vi "Main.vi"() -> ()   [LabVIEW 2018]
uses:
  Typedefs/States.ctl
  Typedefs/Element.ctl
  Typedefs/TestSequence.ctl
  C:/GIT/gaialabviewclient/Gaia_LabVIEW/Resources/JOT.GaiaClient.dll
  Resources/JOT.GaiaClient.dll
panel:
  out "error out":errorcluster
  in  "Exit":bool
  in  "Tab Control":enum32{"TestSequense", "ManualControls"}(tab)
  out "EventLog":string
  in  "StartTest":bool
  in  "DutLock":bool
  in  "BatteryConnector":bool
  # "StateApps"
  # "MainRobot"
  # "More StateApp manual controls \ncan be added here"
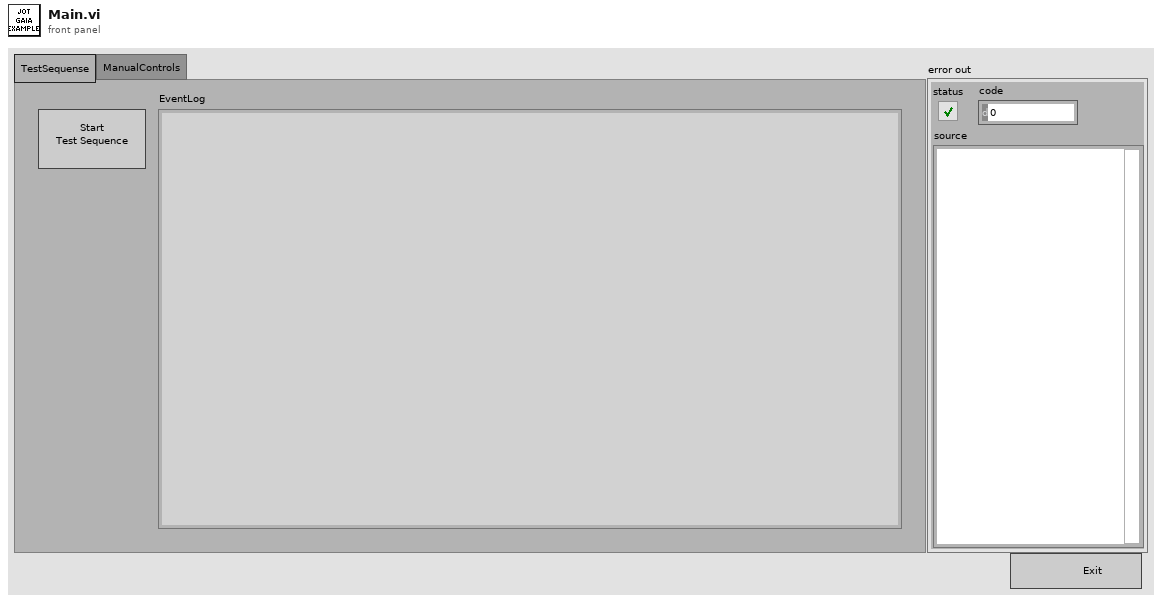
[diagram p1: front panel]
types:
  T1 = typedef "TestSequence.ctl" = enum16{"WaitDUT", "PreliminaryOperations", "WaitSlideClosed", "Test1", "ReleaseDUT"}
  T2 = typedef "Element.ctl" = cluster{"State":T3, "Application":string, "Action":string, "G code":string}
  T3 = typedef "States.ctl" = enum16{"InitGaiaClient", "Idle", "RobotManualCtr", "StateAppsManualCtr", "TestSequence", "Exit"}
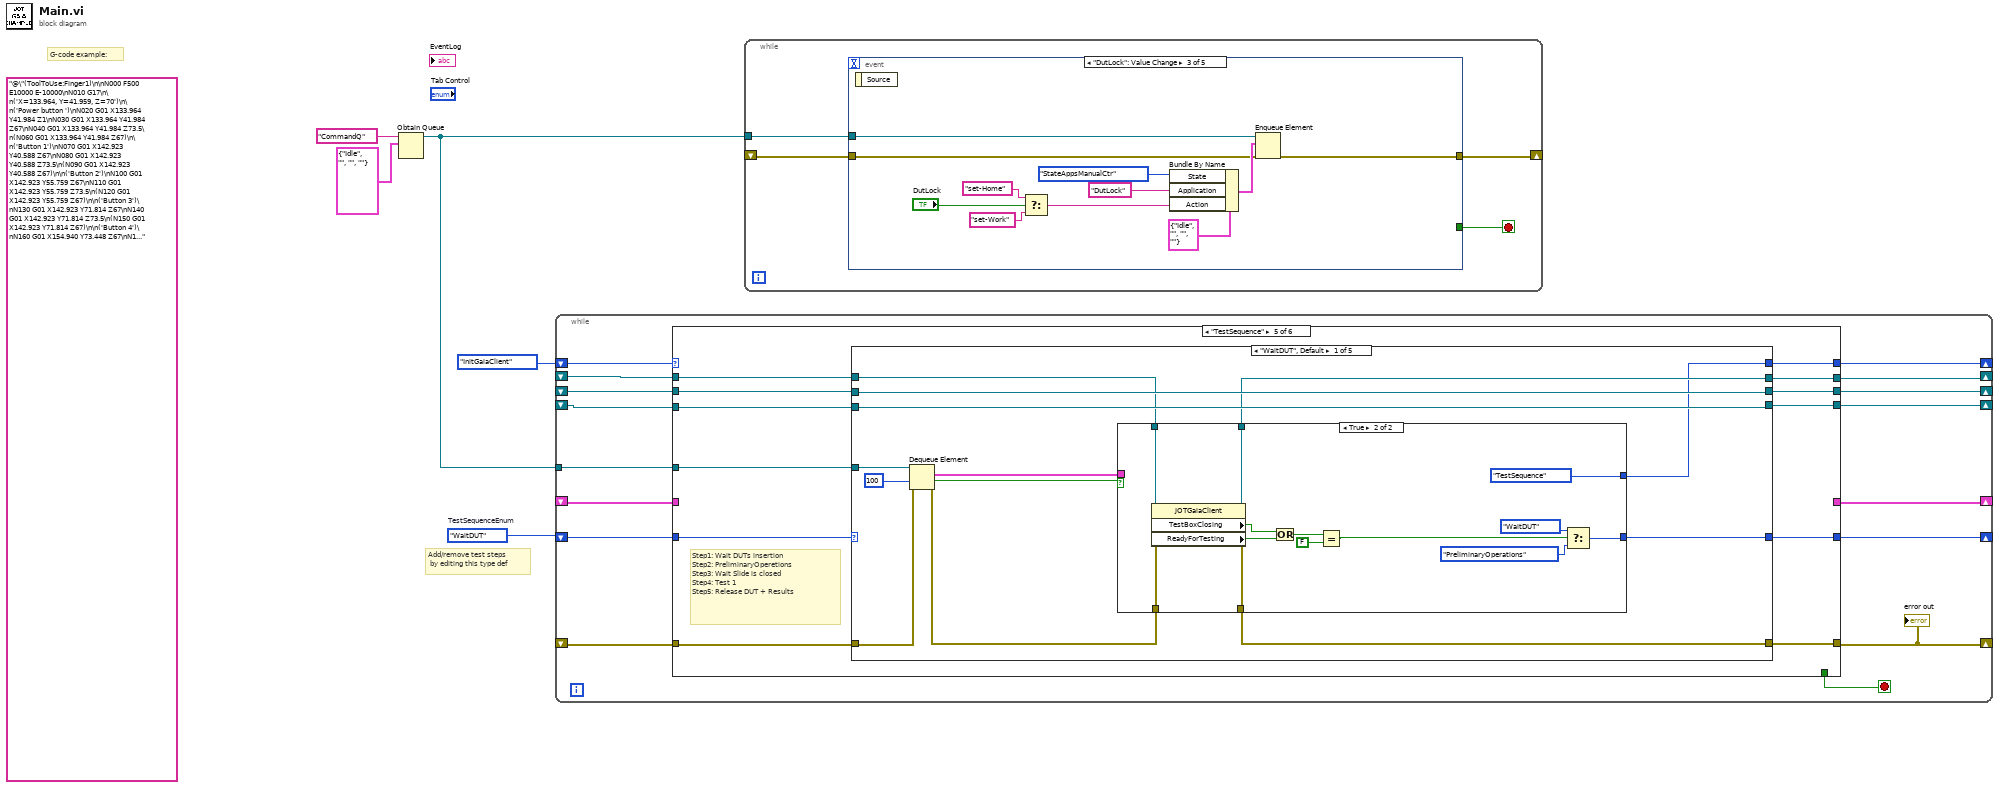
[diagram p0: block diagram]
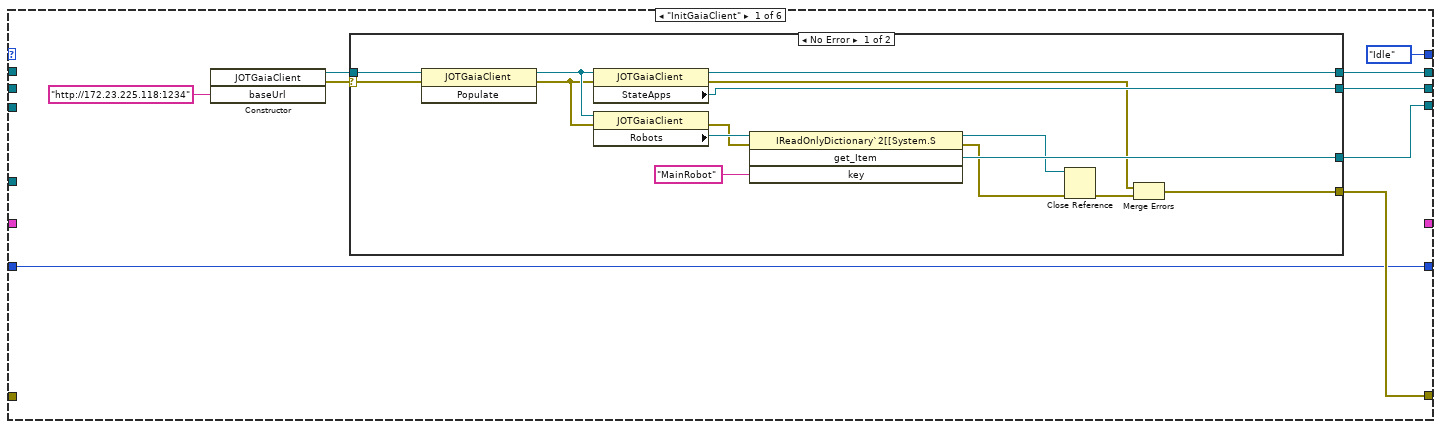
[diagram p2: hidden frame]
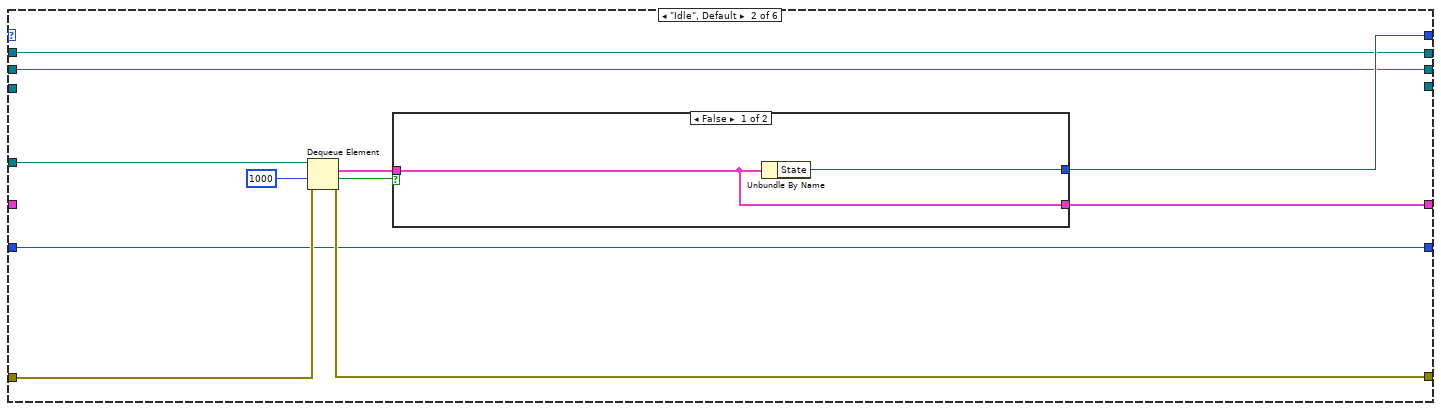
[diagram p4: hidden frame]
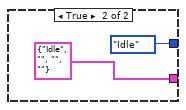
[diagram p5: hidden frame]
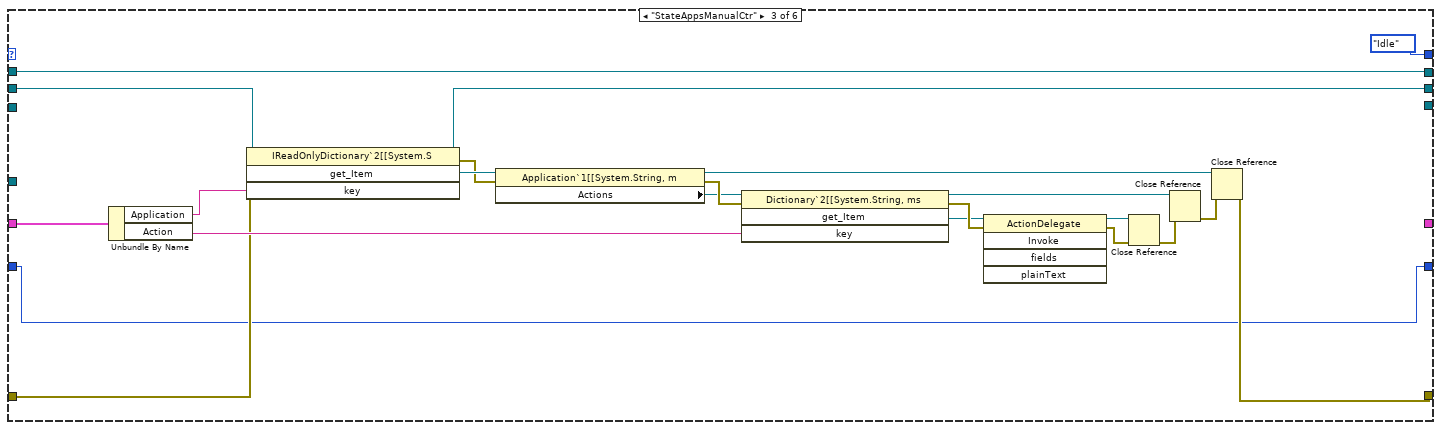
[diagram p6: hidden frame]
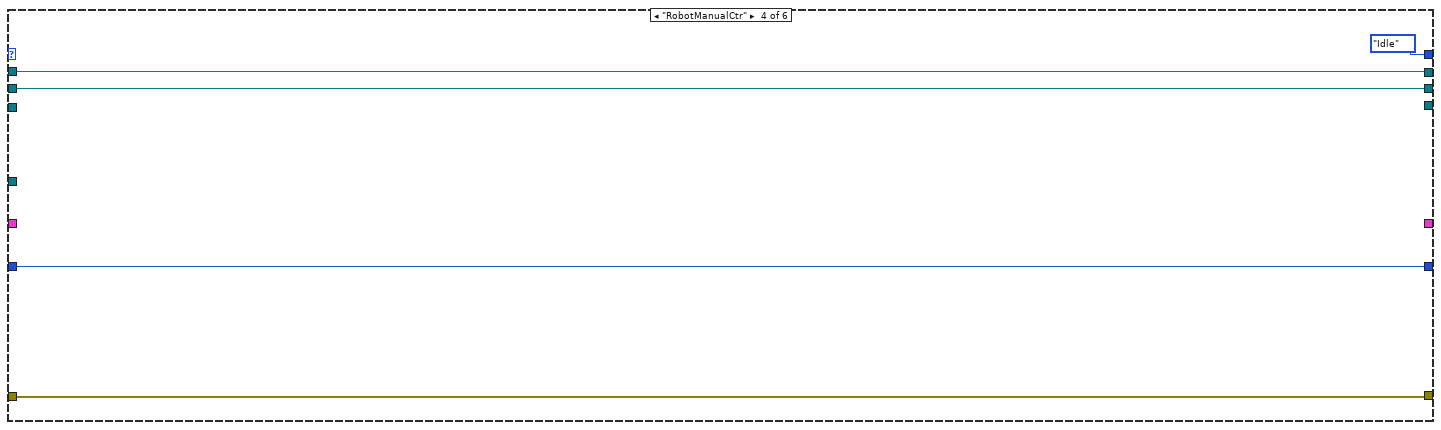
[diagram p7: hidden frame]
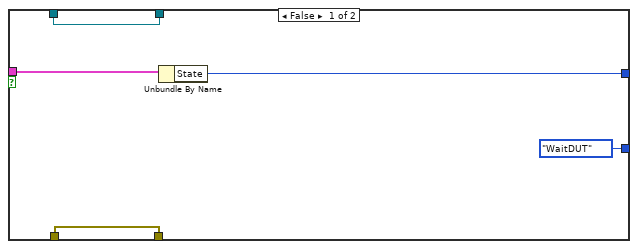
[diagram p8: hidden frame]
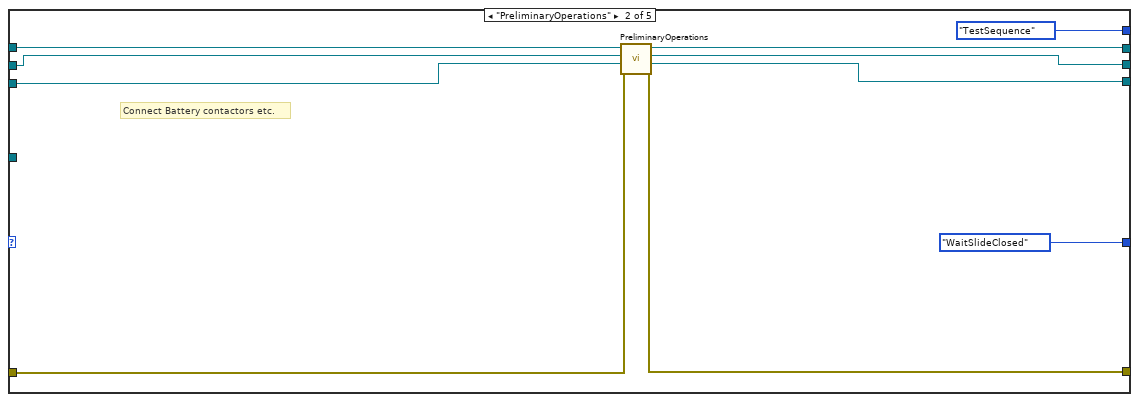
[diagram p9: hidden frame]
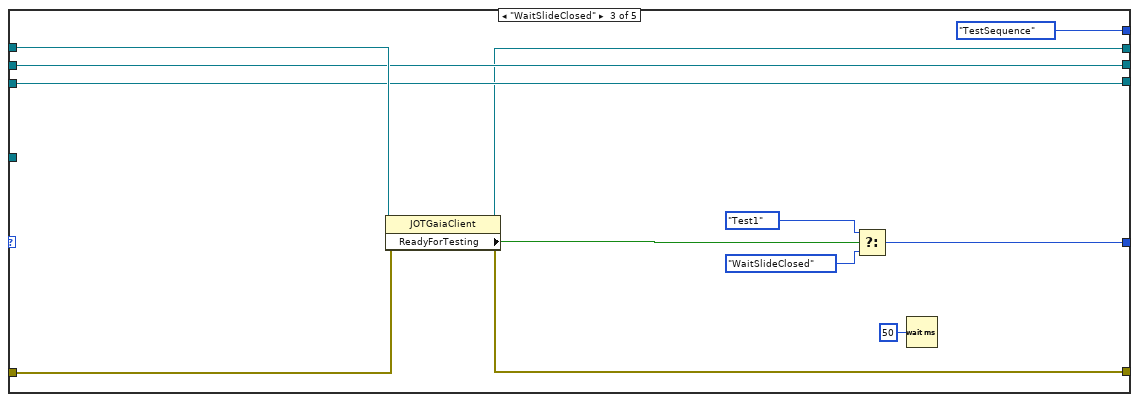
[diagram p10: hidden frame]
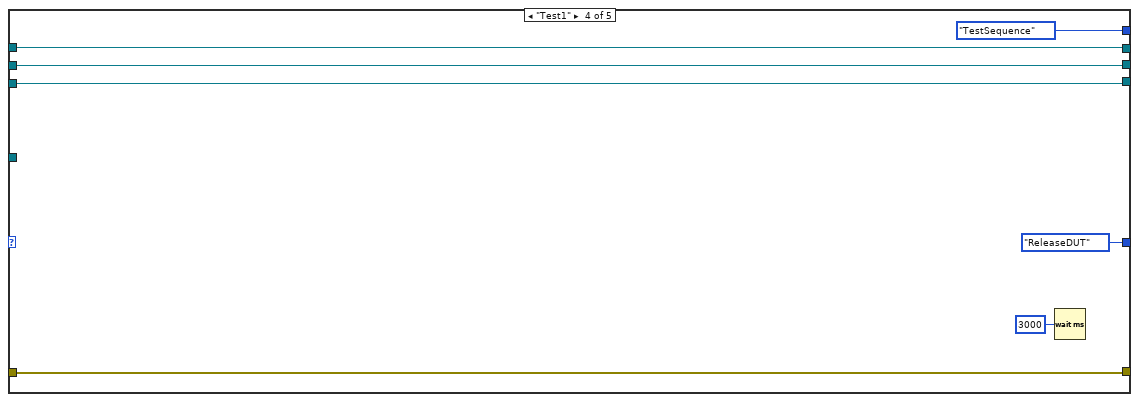
[diagram p11: hidden frame]
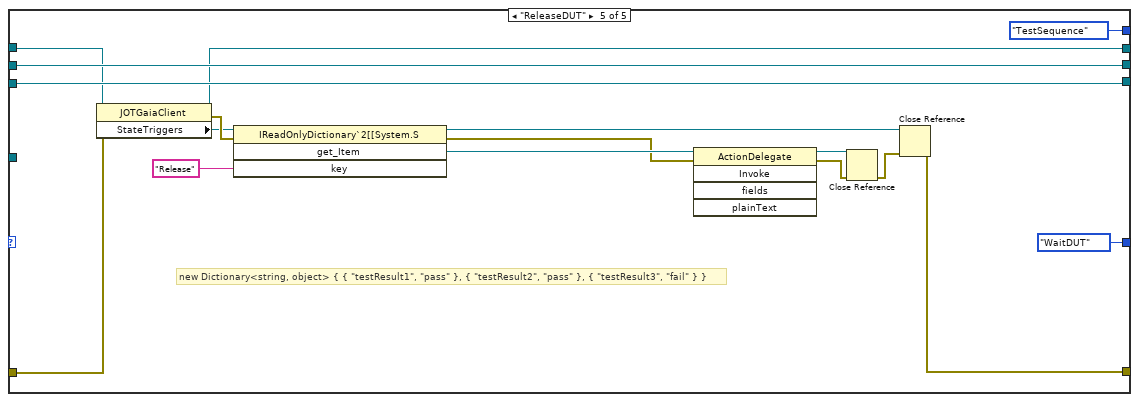
[diagram p12: hidden frame]
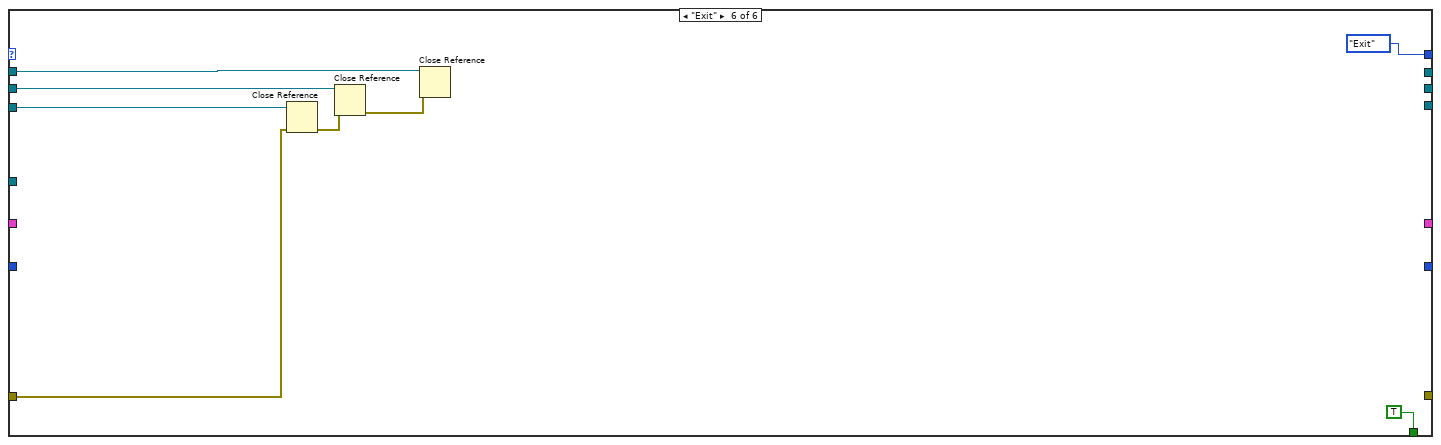
[diagram p13: hidden frame]
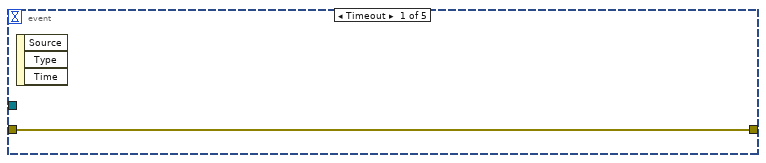
[diagram p14: hidden frame]
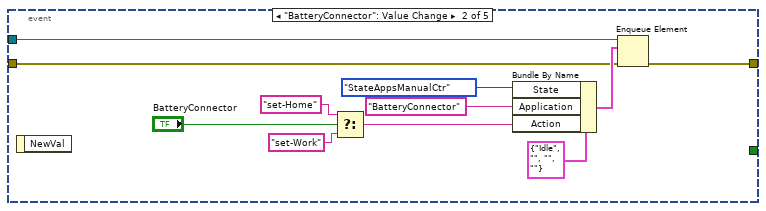
[diagram p15: hidden frame]
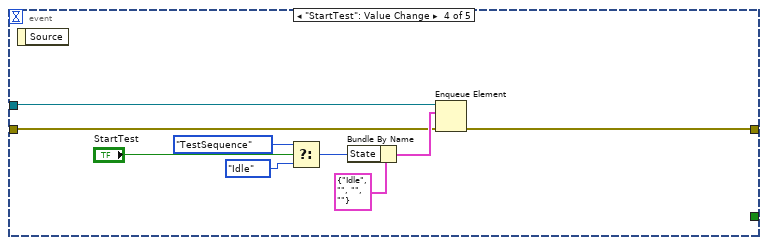
[diagram p16: hidden frame]
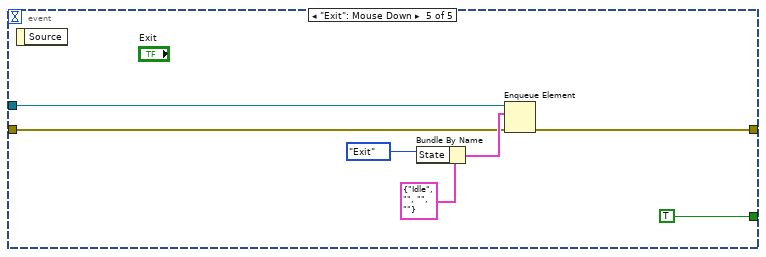
[diagram p17: hidden frame]
diagram:
  w1 = TestSequence."WaitDUT"  # TestSequenceEnum
  (unwired) "@\"(ToolToUse:Finger1)\n\nN000 F500 E10000 E-10000\nN010 G17\n\n('X=133.964, Y=41.959, Z=70')\n\n('Power button ')\nN020 G01 X133.964 Y41.984 Z1\nN030 G01 X133.964 Y41.984 Z67\nN040 G01 X133.964 Y41.984 Z73.5\n(N060 G01 X133.964 Y41.984 Z67)\n\n('Button 1')\nN070 G01 X142.923 Y40.588 Z67\nN080 G01 X142.923 Y40.588 Z73.5\n(N090 G01 X142.923 Y40.588 Z67)\n\n('Button 2')\nN100 G01 X142.923 Y55.759 Z67\nN110 G01 X142.923 Y55.759 Z73.5\n(N120 G01 X142.923 Y55.759 Z67)\n\n('Button 3')\nN130 G01 X142.923 Y71.814 Z67\nN140 G01 X142.923 Y71.814 Z73.5\n(N150 G01 X142.923 Y71.814 Z67)\n\n('Button 4')\nN160 G01 X154.940 Y73.448 Z67\nN170 G01 X154.940 Y73.448 Z73.5\n(N180 G01 X154.940 Y73.448 Z67)\n\n('Button 5')\nN190 G01 X154.940 Y55.778 Z67\nN200 G01 X154.940 Y55.778 Z73.2\n(N210 G01 X154.940 Y55.778 Z67)\n\n('Button 6')\nN220 G01 X154.940 Y38.754 Z67\nN230 G01 X154.940 Y38.754 Z73.5\n(N240 G01 X154.940 Y38.754 Z67)\n\n('Button 7')\nN250 G01 X167.756 Y42.098 Z67\nN260 G01 X167.756 Y42.098 Z73.2\n(N270 G01 X167.756 Y42.098 Z67)\n\n('Button 8')\nN280 G01 X167.756 Y55.883 Z67\nN290 G01 X167.756 Y55.883 Z73.3\n(N300 G01 X167.756 Y55.883 Z67)\n\n('Button 9')\nN310 G01 X167.756 Y69.886 Z67\nN320 G01 X167.756 Y69.886 Z73.2\n(N330 G01 X167.756 Y69.886 Z67)\""
  # "Add/remove test steps\n by editing this type def"
  # "G-code example:"
  n1 = Obtain Queue(name (unnamed)="CommandQ", element data type=T2 {"State"=enum."Idle", "Application"="", "Action"="", "G code"=""}) -> (queue out=w2:refnum<queue>)  [unwired: 3 in, 2 out]
  n2 = while {
    shift-right: [w14] -> _
    shift-left: States."InitGaiaClient" -> [w21]
    shift-right: [w20] -> _
    shift-left: _ -> [w9]
    shift-right: [w19] -> _
    shift-left: _ -> [w8]
    shift-right: [w16] -> _
    shift-left: _ -> [w17]
    shift-right: [w15] -> _
    shift-left: _ -> [w10]
    tunnel: w2 -> [w13]
    shift-right: [w12] -> _
    shift-left: _ -> [w11]
    shift-right: [w6] -> _
    shift-left: w1 -> [w7]
    stop <- w18 stop-if-true
    n3 = case shown="\"TestSequence\"" w21 {
      tunnel: [_ _ _ _ _ TRUE] -> w18
      tunnel: [w28 w48 w62 w85 w95 _] -> w20
      tunnel: [w27 w49 w69 w86 w94 _] -> w19
      tunnel: w17 -> [_ w54 w64 w83 w91 w179]
      tunnel: [w25 w55 w63 w83 w90 _] -> w16
      tunnel: [w26 _ _ _ w96 _] -> w15
      tunnel: [States."Idle" w50 States."Idle" States."Idle" w88 States."Exit"] -> w14
      tunnel: w13 -> [_ w53 _ _ w89 _]
      tunnel: [_ w47 _ _ _ _] -> w12
      tunnel: w11 -> [_ _ w67 _ _ _]
      tunnel: w10 -> [_ _ _ _ w99 w177]
      tunnel: w9 -> [_ w48 w70 w85 w98 w182]
      tunnel: w8 -> [_ w49 w69 w86 w97 w183]
      tunnel: w7 -> [w23 w46 w61 w84 w93 _]
      tunnel: [w23 w46 w61 w84 w92 _] -> w6
      frame "InitGaiaClient" {
        n4 = constructor class="JOTGaiaClient"("baseUrl"="http://172.23.225.118:1234") -> (reference out=w29:refnum<k24>, error out=w22:errorcluster)  [unwired: 3 in, 2 out]
        n5 = case shown="No Error" w22 {
          selector: w22 -> [w31 _]
          tunnel: w29 -> [w45 _]
          tunnel: [w44 _] -> w28
          tunnel: [w43 _] -> w27
          tunnel: [w38 _] -> w26
          tunnel: [w36 _] -> w25
          frame No Error {
            n6 = invoke class="JOTGaiaClient" method="Populate"(reference=w45, error in=w31) -> (reference out=w42:refnum<k24>, error out=w41:errorcluster)  [unwired: 1 in, 1 out]
            n7 = property class="JOTGaiaClient"(reference=w42, error in=w41) -> (reference out=w43:refnum<k24>, error out=w37:errorcluster, "StateApps"=w44:refnum<k24>)
            n8 = property class="JOTGaiaClient"(reference=w42, error in=w41) -> (error out=w39:errorcluster, "Robots"=w40:refnum<k24>)  [unwired: 1 out]
            n9 = invoke class="IReadOnlyDictionary`2[[System.S" method="get_Item"(reference=w40, error in=w39, "key"="MainRobot" ("baseUrl")) -> (reference out=w34:refnum<k24>, error out=w33:errorcluster, "get_Item"=w38:refnum<k24>)  [unwired: 1 in, 1 out]
            n10 = Close Reference(reference=w34, error in (no error)=w33) -> (error out=w32:errorcluster)
            n11 = Merge Errors(w37, w32) -> (w36:errorcluster)
          }
          frame Error {
          }
        }
      }
      frame "Idle", Default {
        n12 = Dequeue Element(queue=w53, timeout in ms (-1)=1000, error in (no error)=w54) -> (element=w56:T2, timed out?=w51:bool, error out=w55:errorcluster)  [unwired: 1 out]
        n13 = case shown="False" w51 {
          tunnel: w56 -> [w57 _]
          tunnel: [w58 States."Idle"] -> w50
          tunnel: [w57 T2 {"State"=enum."Idle", "Application"="", "Action"="", "G code"=""}] -> w47
          frame False {
            n14 = Unbundle By Name(w57) -> ("State"=w58:T3)
          }
          frame True {
          }
        }
      }
      frame "StateAppsManualCtr" {
        n15 = Unbundle By Name(w67) -> ("Application"=w66:string, "Action"=w65:string)
        n16 = invoke class="IReadOnlyDictionary`2[[System.S" method="get_Item"(reference=w70, error in=w64, "key"=w66) -> (reference out=w62:refnum<k24>, error out=w75:errorcluster, "get_Item"=w78:refnum<k24>)  [unwired: 1 in, 1 out]
        n17 = property class="Application`1[[System.String, m"(reference=w78, error in=w75) -> (reference out=w71:refnum<k24>, error out=w79:errorcluster, "Actions"=w76:refnum<k24>)
        n18 = invoke class="Dictionary`2[[System.String, ms" method="get_Item"(reference=w76, error in=w79, "key"=w65) -> (reference out=w82:refnum<k24>, error out=w80:errorcluster, "get_Item"=w77:refnum<k24>)  [unwired: 1 in, 1 out]
        n19 = invoke class="ActionDelegate" method="Invoke"(reference=w77, error in=w80) -> (reference out=w74:refnum<k24>, error out=w81:errorcluster)  [unwired: 3 in, 3 out]
        n20 = Close Reference(reference=w74, error in (no error)=w81) -> (error out=w73:errorcluster)
        n21 = Close Reference(reference=w82, error in (no error)=w73) -> (error out=w72:errorcluster)
        n22 = Close Reference(reference=w71, error in (no error)=w72) -> (error out=w63:errorcluster)
      }
      frame "RobotManualCtr" {
      }
      frame "TestSequence" {
        # "Step1: Wait DUTs insertion\nStep2: PreliminaryOperetions \nStep3: Wait Slide is closed\nStep4: Test 1\nStep5: Release DUT + Results"
        n23 = case shown="\"WaitDUT\", Default" w93 {
          tunnel: w99 -> [w111 w137 w146 w156 w175]
          tunnel: w98 -> [w112 w138 w147 w157 w176]
          tunnel: w97 -> [w110 w139 w152 w158 w171]
          tunnel: [w111 w134 w146 w156 w175] -> w96
          tunnel: [w112 w135 w147 w157 w176] -> w95
          tunnel: [w109 w136 w142 w158 w170] -> w94
          tunnel: [w108 TestSequence."WaitSlideClosed" w149 TestSequence."ReleaseDUT" TestSequence."WaitDUT"] -> w92
          tunnel: w91 -> [w104 w133 w145 w159 w172]
          tunnel: [w107 w132 w144 w159 w160] -> w90
          tunnel: w89 -> [w105 _ _ _ _]
          tunnel: [w102 States."TestSequence" States."TestSequence" States."TestSequence" States."TestSequence"] -> w88
          frame "WaitDUT", Default {
            n24 = Dequeue Element(queue=w105, timeout in ms (-1)=100, error in (no error)=w104) -> (element=w100:T2, timed out?=w101:bool, error out=w103:errorcluster)  [unwired: 1 out]
            n25 = case shown="True" w101 {
              tunnel: w110 -> [w116 w130]
              tunnel: [w116 w129] -> w109
              tunnel: [TestSequence."WaitDUT" w126] -> w108
              tunnel: [w117 w120] -> w107
              tunnel: w103 -> [w117 w119]
              tunnel: [w113 States."TestSequence"] -> w102
              tunnel: w100 -> [w114 _]
              frame False {
                n26 = Unbundle By Name(w114) -> ("State"=w113:T3)
              }
              frame True {
                n27 = property class="JOTGaiaClient"(reference=w130, error in=w119) -> (reference out=w129:refnum<k24>, error out=w120:errorcluster, "TestBoxClosing"=w128:bool, "ReadyForTesting"=w127:bool)
                n28 = Or(x=w128, y=w127) -> (x .or. y?=w123:bool)
                n29 = Equal?(x=w123, y=FALSE) -> (x = y?=w121:bool)
                n30 = Select(t=TestSequence."WaitDUT", s=w121, f=TestSequence."PreliminaryOperations") -> (s? t:f=w126:T1)
              }
            }
          }
          frame "PreliminaryOperations" {
            # "Connect Battery contactors etc."
            n31 = call "PreliminaryOperations.vi"("error IN"=w133, "MainRobotREF_IN"=w137, "StateAppsREF_IN"=w138, "ClientREF_IN"=w139) -> ("error OUT"=w132:errorcluster, "MainRobotREF_OUT"=w134:refnum<k24>, "StateAppsREF_OUT"=w135:refnum<k24>, "ClientREF_OUT"=w136:refnum<k24>)  [unwired: 4 in]
          }
          frame "WaitSlideClosed" {
            n32 = property class="JOTGaiaClient"(reference=w152, error in=w145) -> (reference out=w142:refnum<k24>, error out=w144:errorcluster, "ReadyForTesting"=w143:bool)
            n33 = Select(t=TestSequence."Test1", s=w143, f=TestSequence."WaitSlideClosed") -> (s? t:f=w149:T1)
            n34 = Wait (ms)(milliseconds to wait=u32 50) -> ()  [unwired: 1 out]
          }
          frame "Test1" {
            n35 = Wait (ms)(milliseconds to wait=u32 3000) -> ()  [unwired: 1 out]
          }
          frame "ReleaseDUT" {
            # "new Dictionary<string, object> { { \"testResult1\", \"pass\" }, { \"testResult2\", \"pass\" }, { \"testResult3\", \"fail\" } }"
            n36 = property class="JOTGaiaClient"(reference=w171, error in=w172) -> (reference out=w170:refnum<k24>, error out=w168:errorcluster, "StateTriggers"=w166:refnum<k24>)
            n37 = invoke class="IReadOnlyDictionary`2[[System.S" method="get_Item"(reference=w166, error in=w168, "key"="Release") -> (reference out=w163:refnum<k24>, error out=w165:errorcluster, "get_Item"=w167:refnum<k24>)  [unwired: 1 in, 1 out]
            n38 = invoke class="ActionDelegate" method="Invoke"(reference=w167, error in=w165) -> (reference out=w164:refnum<k24>, error out=w161:errorcluster)  [unwired: 3 in, 3 out]
            n39 = Close Reference(reference=w164, error in (no error)=w161) -> (error out=w162:errorcluster)
            n40 = Close Reference(reference=w163, error in (no error)=w162) -> (error out=w160:errorcluster)
          }
        }
      }
      frame "Exit" {
        n41 = Close Reference(reference=w177, error in (no error)=w179) -> (error out=w180:errorcluster)
        n42 = Close Reference(reference=w182, error in (no error)=w180) -> (error out=w181:errorcluster)
        n43 = Close Reference(reference=w183, error in (no error)=w181) -> ()  [unwired: 1 out]
      }
    }
    "error out" <- w16
  }
  n44 = while {
    tunnel: w2 -> [w188]
    shift-right: [w187] -> _
    shift-left: _ -> [w186]
    stop <- w185 stop-if-true
    n45 = event shown="[2] \"DutLock\": Value Change" {
      selector: _ -> [_ _ _ _ _]
      dyn-events: _ -> [_ _ _ _ _]
      timeout: _ -> [_ _ _ _ _]
      tunnel: w188 -> [_ w193 w211 w217 w223]
      tunnel: [w189 w190 w202 w218 w221] -> w187
      tunnel: w186 -> [w189 w192 w201 w216 w222]
      tunnel: [_ _ _ _ TRUE] -> w185
      event Timeout {
        n46 = event-data() -> ()  [unwired: 1 in, 3 out]
      }
      event "BatteryConnector": Value Change {
        n47 = event-data() -> ()  [unwired: 1 in, 1 out]
        n48 = Select(t="set-Home" ("key"), s="BatteryConnector", f="set-Work" ("key")) -> (s? t:f=w196:string)
        n49 = Bundle By Name(cluster=T2 {"State"=enum."Idle", "Application"="", "Action"="", "G code"=""}, "State"=States."StateAppsManualCtr", "Application"="BatteryConnector", "Action"=w196) -> (w199:T2)
        n50 = Enqueue Element(queue=w193, element=w199, error in (no error)=w192) -> (error out=w190:errorcluster)  [unwired: 1 in, 2 out]
      }
      event "DutLock": Value Change {
        n51 = event-data() -> ()  [unwired: 1 in, 1 out]
        n52 = Select(t="set-Home" ("key"), s="DutLock", f="set-Work" ("key")) -> (s? t:f=w205:string)
        n53 = Bundle By Name(cluster=T2 {"State"=enum."Idle", "Application"="", "Action"="", "G code"=""}, "State"=States."StateAppsManualCtr", "Application"="DutLock", "Action"=w205) -> (w209:T2)
        n54 = Enqueue Element(queue=w211, element=w209, error in (no error)=w201) -> (error out=w202:errorcluster)  [unwired: 1 in, 2 out]
      }
      event "StartTest": Value Change {
        n55 = event-data() -> ()  [unwired: 1 in, 1 out]
        n56 = Select(t=States."TestSequence" ("State"), s="StartTest", f=States."Idle" ("State")) -> (s? t:f=w212:T3)
        n57 = Bundle By Name(cluster=T2 {"State"=enum."Idle", "Application"="", "Action"="", "G code"=""}, "State"=w212) -> (w219:T2)
        n58 = Enqueue Element(queue=w217, element=w219, error in (no error)=w216) -> (error out=w218:errorcluster)  [unwired: 1 in, 2 out]
      }
      event "Exit": Mouse Down {
        n59 = event-data() -> ()  [unwired: 1 in, 1 out]
        n60 = Bundle By Name(cluster=T2 {"State"=enum."Idle", "Application"="", "Action"="", "G code"=""}, "State"=States."Exit") -> (w225:T2)
        n61 = Enqueue Element(queue=w223, element=w225, error in (no error)=w222) -> (error out=w221:errorcluster)  [unwired: 1 in, 2 out]
      }
    }
  }
